vi "Instrument.Lockin.Read Configuration.vi"(8 "error in (no error)":errorcluster, 11 "Instrument.Lockin":refnum<class "Instrument.Lockin.lvclass">) -> (0 "error out":errorcluster, 2 "Configuration":T1={"Channels: AO"={"AO Amp (V)"=[], "AO DC (V)"=[], "AO f (Hz)"=[], "AO Phase (°)"=[], "Function"=[], "I+"=[], "Sweeping"=[]}, "Channels: Reference"={"REF f (Hz)"=[], "REF phi (°)"=[]}, "REF Filter"={"LP cutoff (Hz)"=0.0, "LP prefilter"=FALSE, "60 Hz prefilter"=FALSE, "order"=0, "TC (s)"=0.0}, "Amplifers"={"offsets"=[], "Gain"=[], "Amplifiers"=enum."Manual"}, "DAQ"={"sampling"={"Fs"=0.0, "#s"=500}, "sample mode"=10178, "buffer size (S)"=0}, "Calibration"={"Cal Info"=[]}, "AI Configuration"=[], "AO Configuration"=[]} {"AO Configuration"."output terminal configuration" items=["Default"=-1, "RSE"=10083, "Differential"=10106, "Pseudodifferential"=12529]; "AI Configuration"."input terminal configuration" items=["default"=-1, "RSE"=10083, "NRSE"=10078, "Differential"=10106, "Pseudodifferential"=12529]; "AI Configuration"."AI.Coupling" items=["AC"=10045, "DC"=10050, "GND"=10066]; "DAQ"."sample mode" items=["Finite Samples"=10178, "Continuous Samples"=10123]; "Channels: AO"."AO f (Hz)" min=0.001 max=10000.0; "Channels: AO"."AO DC (V)" format="%.3p"; "Channels: AO"."AO Amp (V)" format="%.3p"; "Channels: Reference"."REF phi (°)" format="%#_3g"}, 3 "Instrument.Lockin out":refnum<class "Instrument.Lockin.lvclass">)   [LabVIEW 2016, in "Instrument.Lockin.lvclass"]
uses:
  Instrument.Lockin.lvclass
  Typedefs/Instrument.Lockin.Configuration--Cluster.ctl
  Typedefs/AO-cluster.ctl
  Typedefs/AO_Amp-array.ctl
  Typedefs/AO_DC-array.ctl
  Typedefs/AO_f-array.ctl
  Typedefs/AO_phi-array.ctl
  Typedefs/Function-array.ctl
  Typedefs/Function-enum.ctl
  Typedefs/REF-cluster.ctl
  Typedefs/REF_f-array.ctl
  Typedefs/REF_phi-array.ctl
  Typedefs/AmplifierType-enum.ctl
  Typedefs/Sampling.ctl
  Typedefs/Cal Info - Cluster.ctl
  Typedefs/AI.config-array.ctl
  Typedefs/AI.config-cluster.ctl
  Typedefs/AI.coupling-enum.ctl
  Typedefs/446xAI-enum.ctl
  Typedefs/DAQType-enum.ctl
  Typedefs/AO.config-array.ctl
  Typedefs/AO.config-cluster.ctl
  Typedefs/446xAO-enum.ctl
  Instrument.Lockin.lvclass/Instrument.Lockin.ctl
panel:
  # "1"
  # "2"
  # "3"
  # "4"
  # "5"
  # "6"
  # "7"
  # "8"
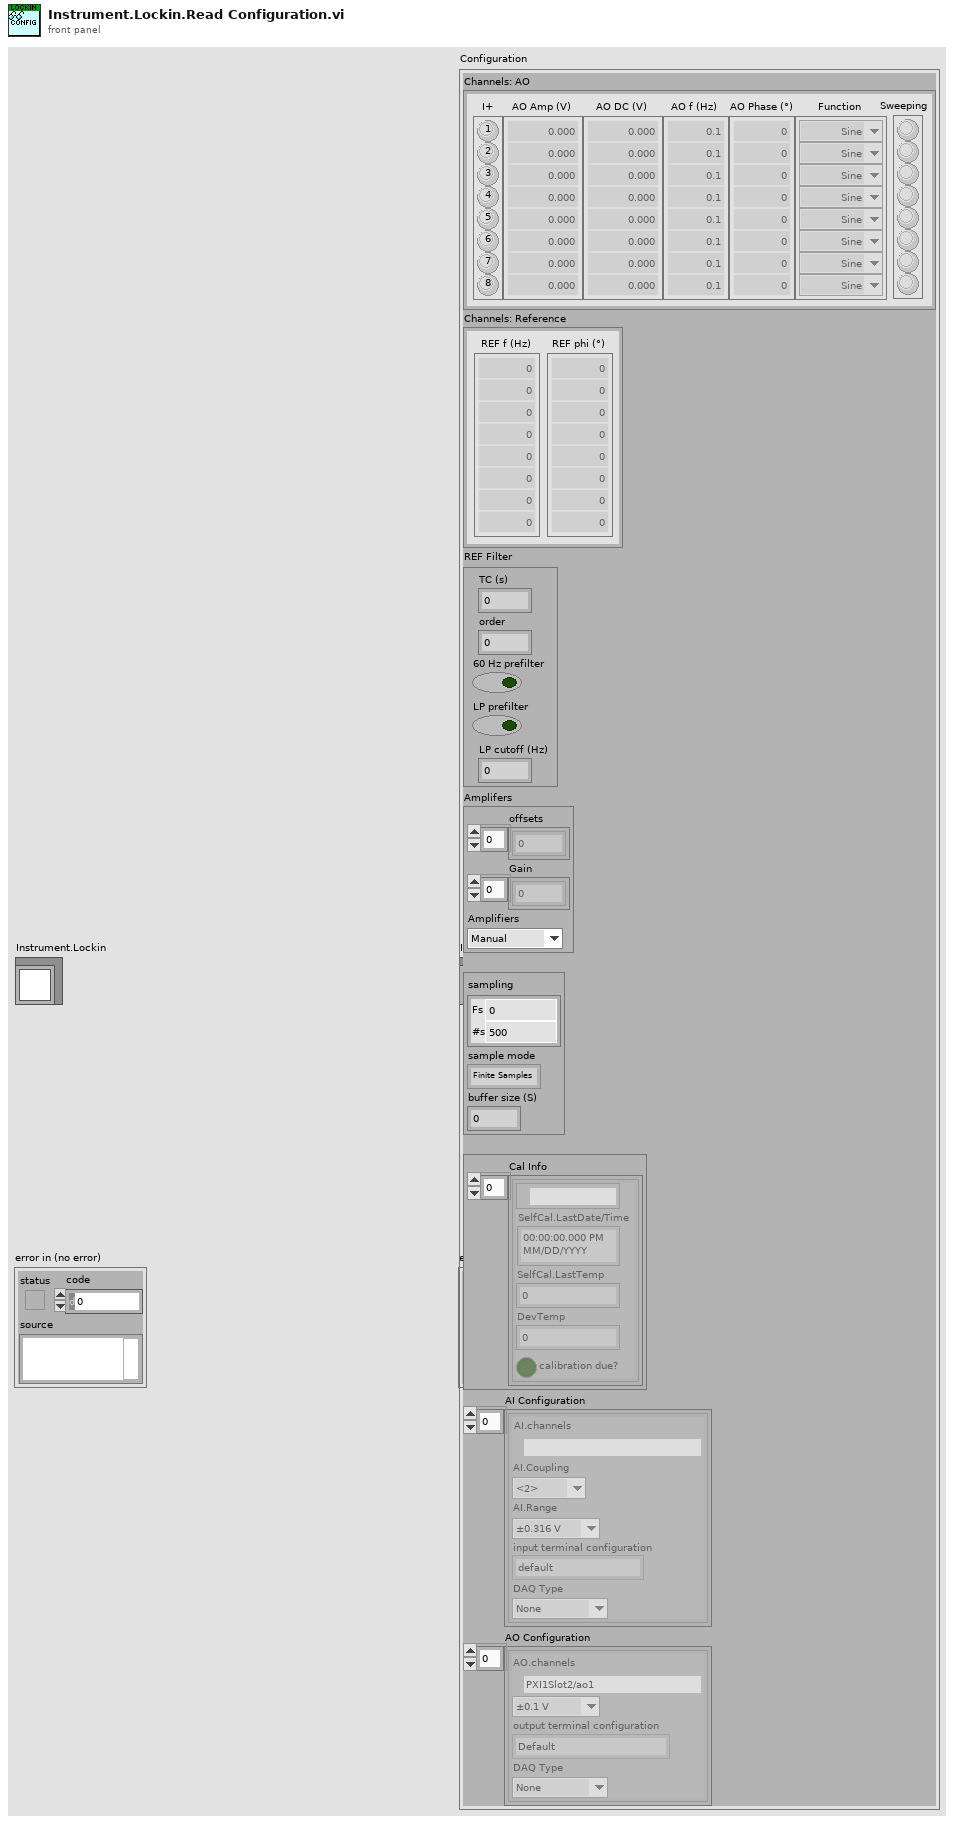
[diagram p1: front panel]
types:
  T1 = typedef "Instrument.Lockin.lvclass/Instrument.Lockin.Configuration--Cluster.ctl" = cluster{"Channels: AO":T2, "Channels: Reference":T9, "REF Filter":cluster{"LP cutoff (Hz)":dbl, "LP prefilter":bool, "60 Hz prefilter":bool, "order":i32, "TC (s)":dbl}, "Amplifers":cluster{"offsets":dbl[], "Gain":dbl[], "Amplifiers":T12}, "DAQ":cluster{"sampling":T13, "sample mode":i32, "buffer size (S)":u32}, "Calibration":cluster{"Cal Info":T14[]}, "AI Configuration":T15, "AO Configuration":T20}
  T2 = typedef "Instrument.Lockin.lvclass/AO-cluster.ctl" = cluster{"AO Amp (V)":T3, "AO DC (V)":T4, "AO f (Hz)":T5, "AO Phase (°)":T6, "Function":T7, "I+":bool[], "Sweeping":bool[]}
  T3 = typedef "Instrument.Lockin.lvclass/AO_Amp-array.ctl" = dbl[]
  T4 = typedef "Instrument.Lockin.lvclass/AO_DC-array.ctl" = dbl[]
  T5 = typedef "Instrument.Lockin.lvclass/AO_f-array.ctl" = dbl[]
  T6 = typedef "Instrument.Lockin.lvclass/AO_phi-array.ctl" = dbl[]
  T7 = typedef "Instrument.Lockin.lvclass/Function-array.ctl" = T8[]
  T8 = typedef "Instrument.Lockin.lvclass/Function-enum.ctl" = enum16{"Sine", "Triangle", "Square", "Sawtooth"}
  T9 = typedef "Instrument.Lockin.lvclass/REF-cluster.ctl" = cluster{"REF f (Hz)":T10, "REF phi (°)":T11}
  T10 = typedef "Instrument.Lockin.lvclass/REF_f-array.ctl" = dbl[]
  T11 = typedef "Instrument.Lockin.lvclass/REF_phi-array.ctl" = dbl[]
  T12 = typedef "Instrument.Lockin.lvclass/AmplifierType-enum.ctl" = enum16{"Manual", "Krohn Hite", "Femto"}
  T13 = typedef "Instrument.Lockin.lvclass/Sampling.ctl" = cluster{"Fs":dbl, "#s":i32}
  T14 = typedef "Instrument.Lockin.lvclass/Cal Info - Cluster.ctl" = cluster{"Active Device":tag, "SelfCal.LastDate/Time":timestamp, "SelfCal.LastTemp":dbl, "DevTemp":dbl, "calibration due?":bool}
  T15 = typedef "Instrument.Lockin.lvclass/AI.config-array.ctl" = T16[]
  T16 = typedef "Instrument.Lockin.lvclass/AI.config-cluster.ctl" = cluster{"AI.channels":tag, "AI.Coupling":T17, "AI.Range":T18, "input terminal configuration":i32, "DAQ Type":T19}
  T17 = typedef "Instrument.Lockin.lvclass/AI.coupling-enum.ctl" = u16
  T18 = typedef "Instrument.Lockin.lvclass/446xAI-enum.ctl" = enum16{"±0.316 V", "±1.00 V", "±3.16 V", "±10.0 V", "±31.6 V", "±42.4 V"}
  T19 = typedef "Instrument.Lockin.lvclass/DAQType-enum.ctl" = enum16{"None", "USB 4431", "PXI 446x"}
  T20 = typedef "Instrument.Lockin.lvclass/AO.config-array.ctl" = T21[]
  T21 = typedef "Instrument.Lockin.lvclass/AO.config-cluster.ctl" = cluster{"AO.channels":tag, "AO.Range":T22, "output terminal configuration":i32, "DAQ Type":T19}
  T22 = typedef "Instrument.Lockin.lvclass/446xAO-enum.ctl" = enum16{"±0.1 V", "±1.0 V", "±10.0 V"}
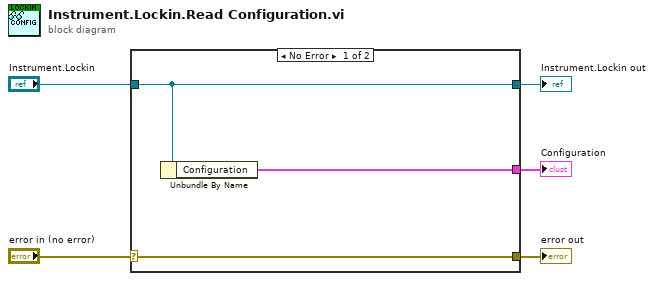
[diagram p0: block diagram]
diagram:
  n1 = case shown="No Error" "error in (no error)" {
    selector: "error in (no error)" -> [w8 w9]
    tunnel: [w8 w9] -> w4
    tunnel: [w7 w10] -> w2
    tunnel: "Instrument.Lockin" -> [w7 w10]
    tunnel: [w6 _] -> w1
    frame No Error {
      n2 = Unbundle By Name(w7) -> ("Configuration"=w6:T1)
    }
    frame Error {
    }
  }
  "error out" <- w4
  "Instrument.Lockin out" <- w2
  "Configuration" <- w1
